vi "Export2CSV.vi"(8 "进度数值":refnum<vi>, 9 "Slide输入":refnum<vi>, 10 "波形数组":cluster{dbl[], dbl[]}[](array[cluster]), 11 "信号名数组":string[](array[string])) -> ()   [LabVIEW 2015]
uses:
  <vilib>/Utility/file.llb/Write Delimited Spreadsheet (string).vi
panel:
  # "正在导出至EXCEL，请稍等"
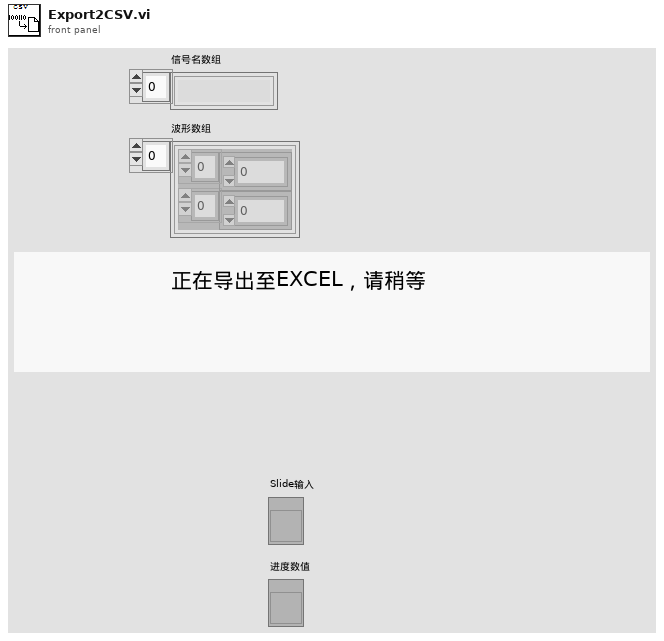
[diagram p1: front panel]
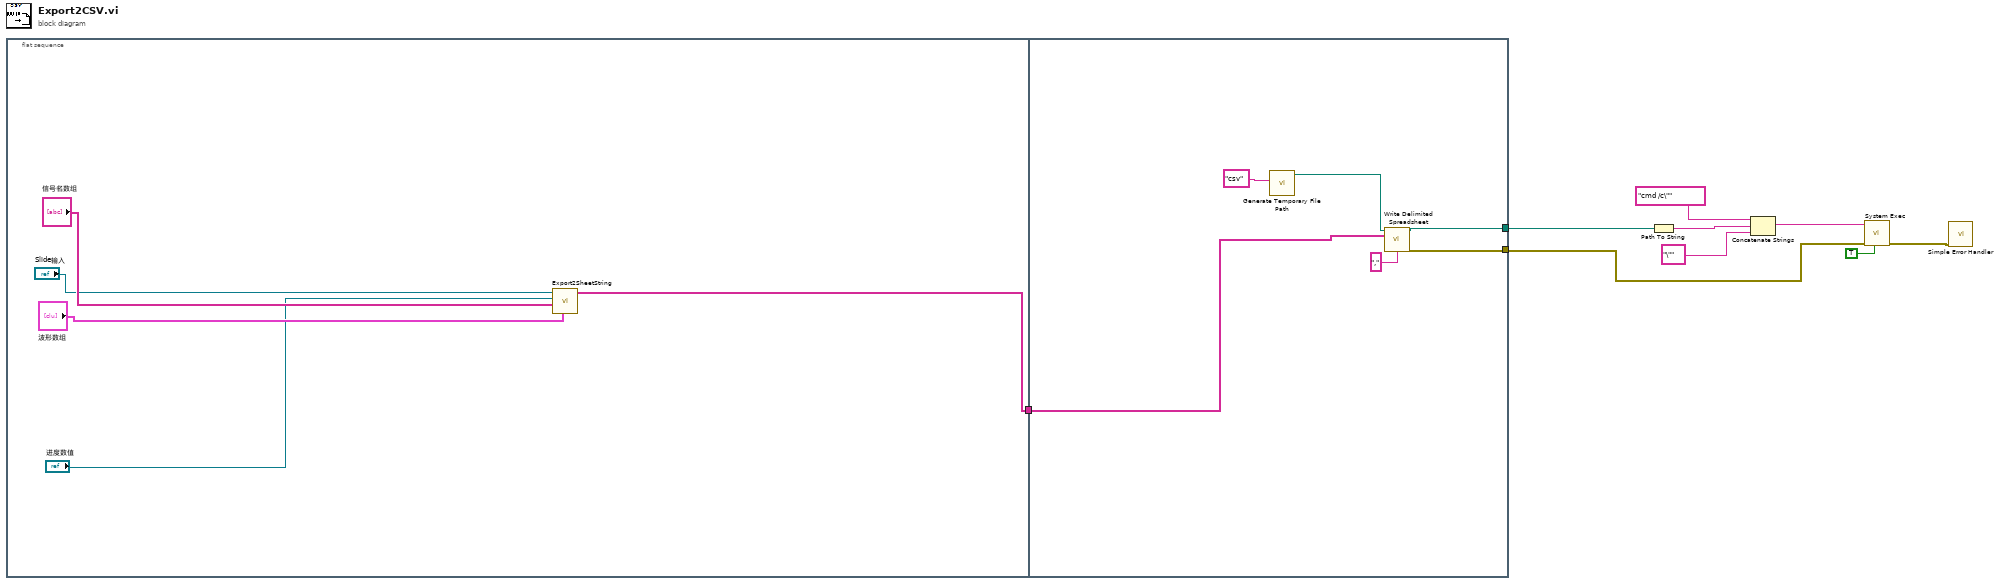
[diagram p0: block diagram]
diagram:
  n1 = flat-sequence {
    tunnel: [w12] -> w9
    tunnel: w9 -> [w18]
    tunnel: [w16] -> w4
    tunnel: [w15] -> w3
    frame #0 {
      n2 = call "Export2SheetString.vi"("波形数组"="波形数组", "信号名数组"="信号名数组", "进度数值"="进度数值", "Slide输入"="Slide输入") -> ("SheetSpread"=w12:string[][])  [unwired: 7 in]
    }
    frame #1 {
      n3 = call <vilib>:"Generate Temporary File Path.vi"("Temporary File Extension (tmp)"="csv") -> ("Unique Temporary File Path"=w17:path)  [unwired: 9 in, 1 out]
      n4 = call-poly <vilib>:"Write Delimited Spreadsheet.vi"("file path (dialog if empty)"=w17, "2D data"=w18, "delimiter (\\t)"="," ("delimiter (\\t)")) -> ("new file path (Not A Path if cancelled)"=w16:path, "error out"=w15:errorcluster)  [unwired: 11 in]
    }
  }
  n5 = Path To String(path=w4) -> (string=w8:string)
  n6 = Concatenate Strings("cmd /c\"" ("字符串"), w8, "\"" ("字符串")) -> (w5:string)
  n7 = call <vilib>:"System Exec.vi"("run minimized? (F)"=TRUE, "error in (no error)"=w3, "command line"=w5) -> ("error out"=w2:errorcluster)  [unwired: 5 in, 3 out]
  n8 = call <vilib>:"Simple Error Handler.vi"("error in (no error)"=w2) -> ()  [unwired: 4 in, 5 out]
